vi "Destroy Main DataTransfer Queues.vi"(8 "error in (no error)":errorcluster, 11 "Main in":refnum<class "Main.lvclass">) -> (0 "error out":errorcluster, 3 "Main out":refnum<class "Main.lvclass">)   [LabVIEW 2019, in "Main.lvclass"]
doc: "Developed by Kevin Thompson\nkevin@thompsonengineering.net\n\nCopyright 2020\nThompson Engineering, LLC"
uses:
  Main.lvclass
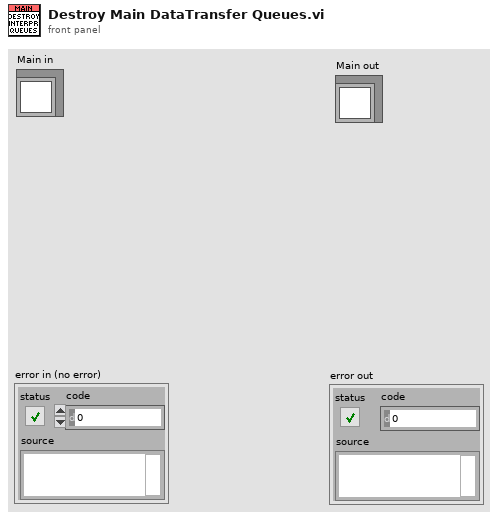
[diagram p1: front panel]
types:
  T1 = typedef "InverterWaveforms--QRef.ctl" = refnum<queue>
  T2 = typedef "DataProcAuxDat--Qref.ctl" = refnum<queue>
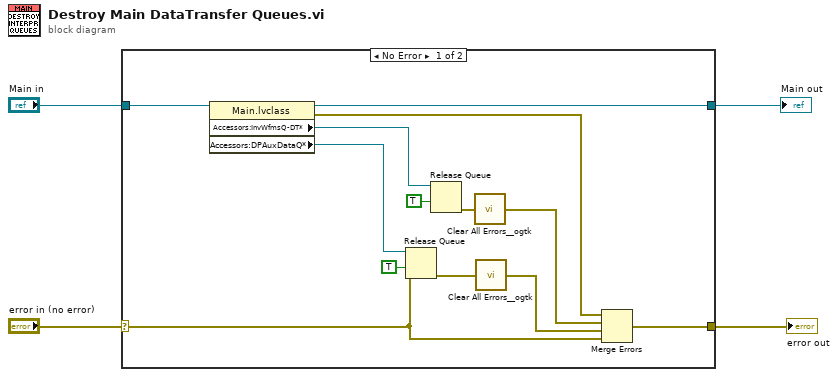
[diagram p0: block diagram]
diagram:
  n1 = case shown="No Error" "error in (no error)" {
    selector: "error in (no error)" -> [w7 w19]
    tunnel: [w15 w19] -> w4
    tunnel: "Main in" -> [w17 w18]
    tunnel: [w16 w18] -> w1
    frame No Error {
      n2 = property class="Main.lvclass"(reference=w17) -> (reference out=w16:refnum<class "Main.lvclass">, error out=w14:errorcluster, "Accessors:InvWfmsQ-DT*"=w11:T1, "Accessors:DPAuxDataQ*"=w12:T2)  [unwired: 1 in]
      n3 = Release Queue(queue=w12, force destroy? (F)=TRUE, error in (no error)=w7) -> (error out=w8:errorcluster)  [unwired: 2 out]
      n4 = Release Queue(queue=w11, force destroy? (F)=TRUE) -> (error out=w13:errorcluster)  [unwired: 1 in, 2 out]
      n5 = call <userlib>:"Clear All Errors__ogtk.vi"("Error In"=w13) -> ("Error Out"=w6:errorcluster)  [unwired: 3 in]
      n6 = call <userlib>:"Clear All Errors__ogtk.vi"("Error In"=w8) -> ("Error Out"=w5:errorcluster)  [unwired: 3 in]
      n7 = Merge Errors(w14, w6, w5, w7) -> (w15:errorcluster)
    }
    frame Error {
    }
  }
  "error out" <- w4
  "Main out" <- w1
